vi "45 deg slice.vi"() -> ()   [LabVIEW 2020]
uses:
  <userlib>/_OpenG.lib/array/array.llb/Sort 1D Array (String)__ogtk.vi
  <resource>/objmgr/IMAQImage.rc
  <vilib>/vision/NI_Vision_Development_Module.lvlib
panel:
  out "Selected Plane 2":T1(plugin-control)
  in  "3D options":T2={"alpha"=30.0, "beta"=30.0, "border"=20, "background"=85, "plane"=2} {"beta" min=15 max=45 format="%.2f"; "alpha" min=15 max=45 format="%.2f"}
  in  "X scaling (times)":i32=1
  in  "Axis":enum16{"X-Projection", "Y-Projection"}(ring)
  out "-45 degrees":T1(plugin-control)
  out "Index of miniscan to be extracted from each plane":i32[](array[numeric])
  out "Selected Plane":T1(plugin-control)
  out "+45 degrees":T1(plugin-control)
  in  "Plane":i32=50 min=1
  in  "Demo files folder":path=path "C:/Users/Theo/Desktop/140610_11_10_21"
  out "Number of images":i32=34
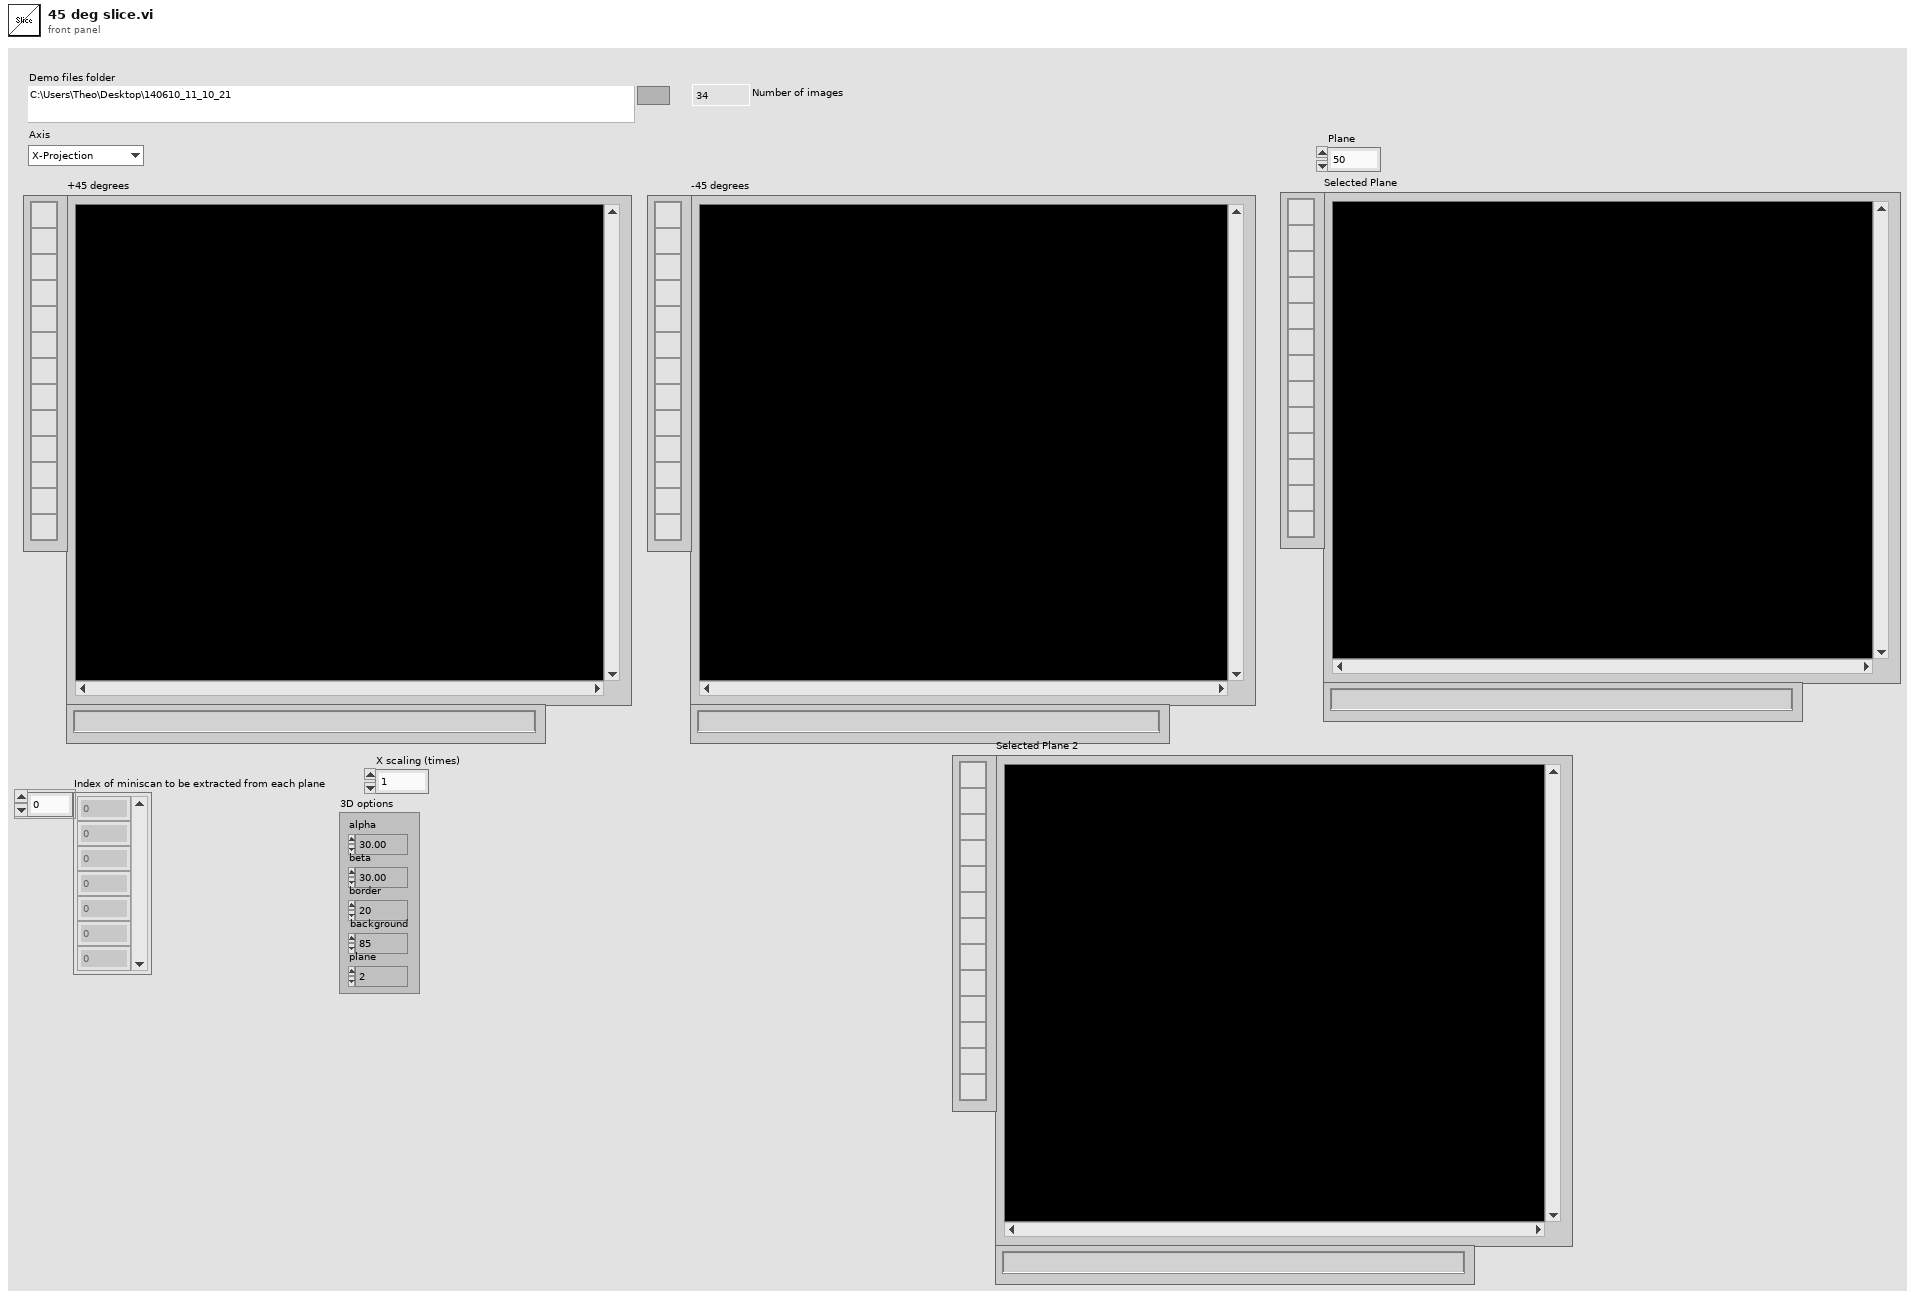
[diagram p1: front panel]
types:
  T1 = typedef "IMAQ Image.ctl" = refnum<image>
  T2 = cluster{"alpha":sgl, "beta":sgl, "border":i32, "background":i32, "plane":i32}
  T3 = typedef "Image Type" = u32
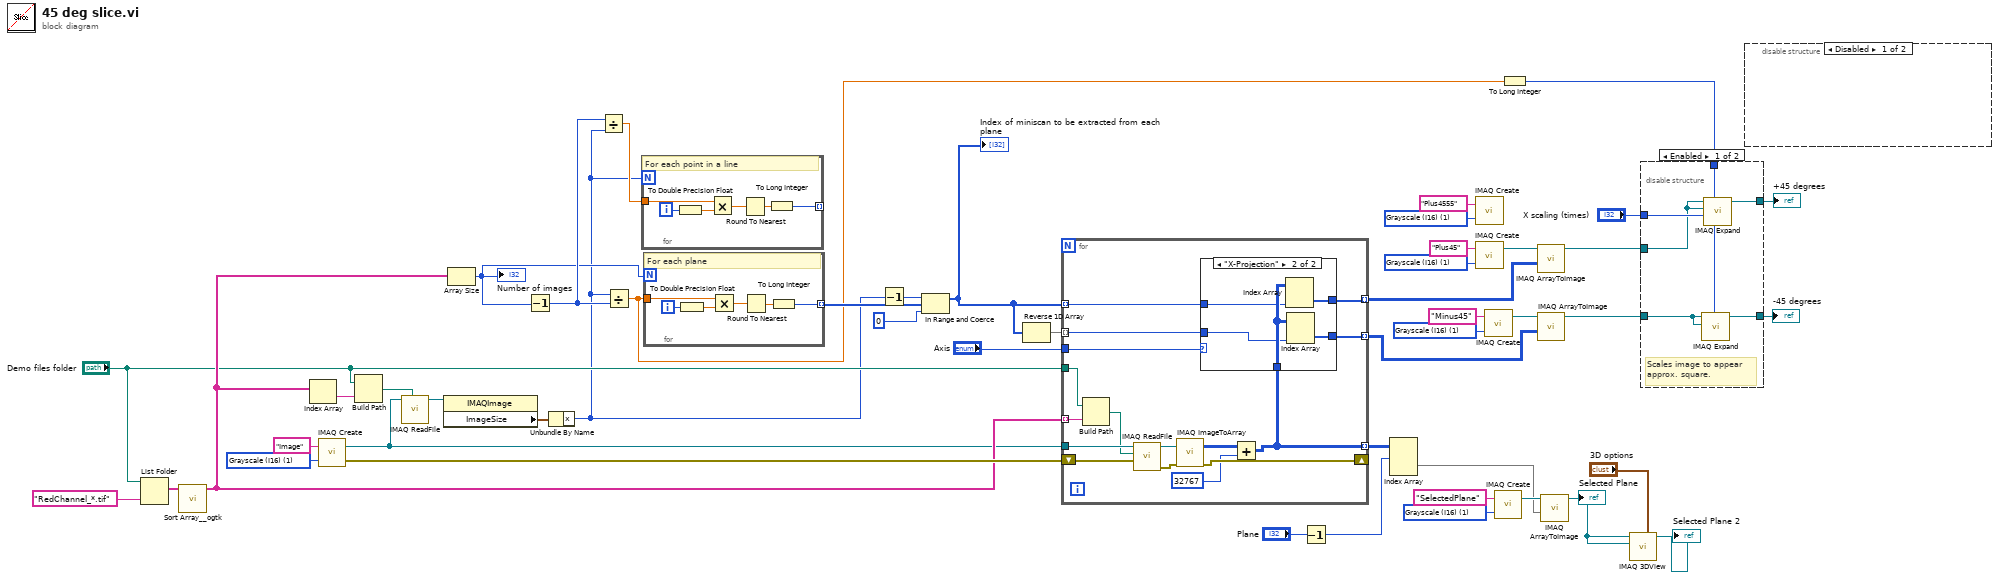
[diagram p0: block diagram]
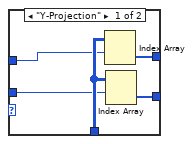
[diagram p4: hidden frame]
diagram:
  w11 = T3 1 items=["Grayscale (U8)", "Grayscale (I16)", "Grayscale (SGL)", "Complex (CSG)", "RGB (U32)", "HSL (U32)", "RGB (U64)", "Grayscale (U16)"] ("Image Type")
  w15 = T3 1 items=["Grayscale (U8)", "Grayscale (I16)", "Grayscale (SGL)", "Complex (CSG)", "RGB (U32)", "HSL (U32)", "RGB (U64)", "Grayscale (U16)"] ("Image Type")
  w30 = T3 1 items=["Grayscale (U8)", "Grayscale (I16)", "Grayscale (SGL)", "Complex (CSG)", "RGB (U32)", "HSL (U32)", "RGB (U64)", "Grayscale (U16)"] ("Image Type")
  w35 = T3 1 items=["Grayscale (U8)", "Grayscale (I16)", "Grayscale (SGL)", "Complex (CSG)", "RGB (U32)", "HSL (U32)", "RGB (U64)", "Grayscale (U16)"] ("Image Type")
  w47 = T3 1 items=["Grayscale (U8)", "Grayscale (I16)", "Grayscale (SGL)", "Complex (CSG)", "RGB (U32)", "HSL (U32)", "RGB (U64)", "Grayscale (U16)"] ("Image Type")
  n1 = List Folder(path="Demo files folder", pattern="RedChannel_*.tif") -> (filenames=w45:string[])  [unwired: 2 in, 3 out]
  n2 = call-poly <userlib>:"Sort Array__ogtk.vi"("Array in"=w45) -> ("Sorted Array out"=w43:string[])  [unwired: 9 in, 1 out]
  n3 = Index Array(array=w43) -> (element=w41:string)  [unwired: 1 in]
  n4 = call "IMAQ Create"("Image Name"="Image", "Image Type"=w47) -> ("New Image"=w40:T1, "error out"=w46:errorcluster)  [unwired: 3 in]
  n5 = Build Path(base path="Demo files folder", name or relative path=w41) -> (appended path=w39:path)
  n6 = call "IMAQ ReadFile"("File Path"=w39, "Image"=w40) -> ("Image Out"=w38:T1)  [unwired: 5 in, 4 out]
  n7 = property class="IMAQImage"(reference=w38) -> ("ImageSize"=w44:cluster{"x":i32, "y":i32})  [unwired: 1 in, 2 out]
  n8 = Array Size(array=w43) -> (size(s)=w23:i32)
  "Number of images" <- w23
  n9 = Decrement(x=w23) -> (x-1=w33:i32)
  n10 = Unbundle By Name(w44) -> ("x"=w20:i32)
  n11 = Divide(x=w33, y=w20) -> (x/y=w32:dbl)
  n12 = Divide(x=w20, y=w33) -> (x/y=w9:dbl)
  n13 = for {
    N: w20 -> [_]
    tunnel: w32 -> [w54]
    tunnel: [w51] -> _ mode=indexing
    i -> [w52]
    # "For each point in a line"
    n14 = To Double Precision Float(number=w52) -> (double precision float=w50:dbl)
    n15 = Multiply(x=w54, y=w50) -> (x*y=w53:dbl)
    n16 = Round To Nearest(number=w53) -> (nearest integer value=w55:dbl)
    n17 = To Long Integer(number=w55) -> (32bit integer=w51:i32)
  }
  n18 = for {
    N: w23 -> [_]
    tunnel: w9 -> [w60]
    tunnel: [w57] -> w24 mode=indexing
    i -> [w58]
    # "For each plane"
    n19 = To Double Precision Float(number=w58) -> (double precision float=w56:dbl)
    n20 = Multiply(x=w60, y=w56) -> (x*y=w59:dbl)
    n21 = Round To Nearest(number=w59) -> (nearest integer value=w61:dbl)
    n22 = To Long Integer(number=w61) -> (32bit integer=w57:i32)
  }
  n23 = Decrement(x=w20) -> (x-1=w19:i32)
  n24 = In Range and Coerce(upper limit=w19, x=w24, lower limit=0 ("size(s)")) -> (coerced(x)=w21:i32[])  [unwired: 1 out]
  "Index of miniscan to be extracted from each plane" <- w21
  n25 = Reverse 1D Array(array=w21) -> (reversed array=w26:i32[])
  n26 = for {
    tunnel: w40 -> [w77]
    tunnel: "Demo files folder" -> [w76]
    tunnel: w43 -> [w74] mode=indexing
    shift-right: [w73] -> _
    shift-left: w46 -> [w72]
    tunnel: w21 -> [w64] mode=indexing
    tunnel: [w69] -> w18 mode=indexing
    tunnel: [w66] -> w37 mode=indexing
    tunnel: w26 -> [w63] mode=indexing
    tunnel: [w65] -> w14 mode=indexing
    tunnel: "Axis" -> [w62]
    n27 = Build Path(base path=w76, name or relative path=w74) -> (appended path=w75:path)
    n28 = call "IMAQ ReadFile"("File Path"=w75, "error in (no error)"=w72, "Image"=w77) -> ("error out"=w71:errorcluster, "Image Out"=w70:T1)  [unwired: 4 in, 3 out]
    n29 = call "IMAQ ImageToArray"("error in (no error)"=w71, "Image"=w70) -> ("error out"=w73:errorcluster, "Image Pixels (I16)"=w68:i16[][])  [unwired: 2 in, 3 out]
    n30 = Add(x=w68, y=i16 32767) -> (x+y=w66:i16[][])
    n31 = case shown="\"X-Projection\"" w62 {
      tunnel: [w82 w87] -> w69
      tunnel: w66 -> [w81 w86]
      tunnel: [w80 w85] -> w65
      tunnel: w64 -> [w79 w84]
      tunnel: w63 -> [w78 w83]
      frame "Y-Projection" {
        n32 = Index Array(array=w81, index (row)=w79) -> (element=w82:i16[])  [unwired: 1 in]
        n33 = Index Array(array=w81, index (row)=w78) -> (element=w80:i16[])  [unwired: 1 in]
      }
      frame "X-Projection" {
        n34 = Index Array(array=w86, index (col)=w84) -> (element=w87:i16[])  [unwired: 1 in]
        n35 = Index Array(array=w86, index (col)=w83) -> (element=w85:i16[])  [unwired: 1 in]
      }
    }
  }
  n36 = Decrement(x="Plane") -> (x-1=w27:i32)
  n37 = Index Array(array=w37, index (dim 0)=w27) -> (element=w28:i16[][])  [unwired: 2 in]
  n38 = call "IMAQ Create"("Image Name"="Plus4555", "Image Type"=w11) -> ()  [unwired: 3 in, 2 out]
  n39 = call "IMAQ Create"("Image Name"="Plus45", "Image Type"=w35) -> ("New Image"=w25:T1)  [unwired: 3 in, 1 out]
  n40 = call "IMAQ Create"("Image Name"="Minus45", "Image Type"=w15) -> ("New Image"=w17:T1)  [unwired: 3 in, 1 out]
  n41 = call "IMAQ Create"("Image Name"="SelectedPlane", "Image Type"=w30) -> ("New Image"=w29:T1)  [unwired: 3 in, 1 out]
  n42 = To Long Integer(number=w9) -> (32bit integer=w4:i32)
  n43 = call "IMAQ ArrayToImage"("Image Pixels (I16)"=w18, "Image"=w25) -> ("Image Out"=w7:T1)  [unwired: 8 in, 1 out]
  n44 = call "IMAQ ArrayToImage"("Image Pixels (I16)"=w14, "Image"=w17) -> ("Image Out"=w6:T1)  [unwired: 8 in, 1 out]
  n45 = call "IMAQ ArrayToImage"("Image Pixels (I16)"=w28, "Image"=w29) -> ("Image Out"=w2:T1)  [unwired: 8 in, 1 out]
  "Selected Plane" <- w2
  n46 = call "IMAQ 3DView"("3D options"="3D options", "Image Dst"=w2, "Image Src"=w2) -> ("Image Dst Out"=→"Selected Plane 2":T1)  [unwired: 7 in, 1 out]
  n47 = disable-structure shown="Enabled" {
    disable-tunnel: "X scaling (times)" -> [w93 _]
    disable-tunnel: [w92 w95] -> w8
    disable-tunnel: w7 -> [w91 w95]
    disable-tunnel: w6 -> [w90 w94]
    disable-tunnel: [w89 w94] -> w5
    disable-tunnel: w4 -> [w88 _]
    frame Enabled {
      # "Scales image to appear\napprox. square."
      n48 = call "IMAQ Expand"("Y Duplication Step"=w88, "Image Dst"=w90, "Image Src"=w90) -> ("Image Dst Out"=w89:T1)  [unwired: 7 in, 1 out]
      n49 = call "IMAQ Expand"("Y Duplication Step"=w88, "X Duplication Step"=w93, "Image Dst"=w91, "Image Src"=w91) -> ("Image Dst Out"=w92:T1)  [unwired: 6 in, 1 out]
    }
    frame Disabled {
    }
  }
  "-45 degrees" <- w5
  "+45 degrees" <- w8
  n50 = disable-structure shown="Disabled" {
    frame Disabled {
    }
    frame Enabled {
    }
  }
